vi "Create Channel Arbitrary Waveform I32 [ACH] Core.vi"(8 "error in (no error)":errorcluster, 9 "Waveform Data Array":i32[](array[numeric]) caption="waveform data array", 10 "Channel Name (\"\")":string="CHANNEL1" caption="channel name (\"CHANNEL1\")", 11 "IVI_Fgen in":refnum<class "IVI_Fgen.lvclass">) -> (0 "error out":errorcluster, 2 "waveform handle":i32, 3 "IVI_Fgen out":refnum<class "IVI_Fgen.lvclass">)   [LabVIEW 2013, in "IVI_Fgen.lvlib" / "IVI_Fgen.lvclass"]
doc: "This VI creates a channel-specific arbitrary waveform and returns a handle that identifies that waveform. Data is passed in as 32-bit binary data. If the arbitrary waveform generator supports formats smaller than 32 bits, read the IviFgen Binary Alignment [AB] property to determine whether to left or right justify the data before passing it to this call. \n\nYou pass this handle to the IviFgen Configure Arbitrary Waveform [ARB] VI to produce that waveform. You also use the handles this VI returns to specify a sequence of arbitrary waveforms with the IviFgen Create Arbitrary Sequence [SEQ] VI.\n\nIf the instrument does not support channel-based arbitrary waveform creation, use IviFgen Create Arbitrary Waveform VI.\n\nUse the IviFgen Create Channel Arbitrary Waveform Int16 [AB] VI to create a channel-specific arbitrary waveform if you want to pass data in 16-bit binary. Use the IviFgen Create Channel Arbitrary Waveform [ACH] VI to create a channel-specific arbitrary waveform with normalized data.\n\nNote:\n\n(1) This VI is part of the IviFgenArbWfmBinary [AB] extension group."
uses:
  IVI_Fgen.lvclass
  IVI_Fgen.lvclass/IVI_Fgen.ctl
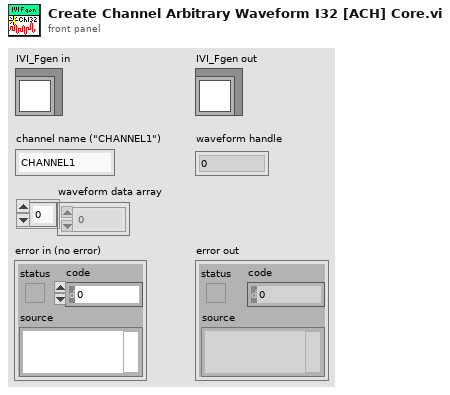
[diagram p1: front panel]
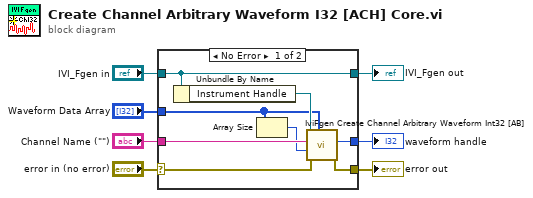
[diagram p0: block diagram]
diagram:
  n1 = case shown="No Error" "error in (no error)" {
    selector: "error in (no error)" -> [w13 w17]
    tunnel: [w12 w17] -> w6
    tunnel: [w15 w16] -> w4
    tunnel: "IVI_Fgen in" -> [w15 w16]
    tunnel: "Waveform Data Array" -> [w8 _]
    tunnel: [w11 _] -> w2
    tunnel: "Channel Name (\"\")" -> [w10 _]
    frame No Error {
      n2 = Unbundle By Name(w15) -> ("Instrument Handle"=w14:refnum<k15>)
      n3 = Array Size(array=w8) -> (size(s)=w9:i32)
      n4 = call <vilib>:"IviFgen Create Channel Arbitrary Waveform Int32 [AB].vi"("Waveform Data Array"=w8, "error in (no error)"=w13, "Waveform Size"=w9, "Channel Name (\"\")"=w10, "instrument handle"=w14) -> ("error out"=w12:errorcluster, "Waveform Handle"=w11:i32)  [unwired: 4 in, 1 out]
    }
    frame Error {
    }
  }
  "error out" <- w6
  "IVI_Fgen out" <- w4
  "waveform handle" <- w2
